vi "XYZ_XYStage.vi"(0 "command":string, 5 "XY details":string, 7 "VISA Write_Read":T1={"VISA resource name"="", "instrument model"="XY-STAGE:MODEL", "command array"=[], "command terminator"="\r", "expected reply"="\r", "reply terminator"="\r", "numeric array out"=[], "string array out"=[]}, 11 "Error in (no error)":errorcluster) -> (4 "x":dbl, 6 "y":dbl, 8 "Success":bool, 10 "VISA Write_Read out":T1={"VISA resource name"="", "instrument model"="XY-STAGE:MODEL", "command array"=[], "command terminator"="\r", "expected reply"="\r", "reply terminator"="\r", "numeric array out"=[], "string array out"=[]}, 15 "Error out":errorcluster)   [LabVIEW 2013]
uses:
  TypeDef VISA Write_Read.ctl
  <vilib>/Instr/_visa.llb/VISA Flush IO Buffer Mask.ctl
  Global.vi
  <vilib>/Instr/_visa.llb/VISA Configure Serial Port (Instr).vi
panel:
  in  "VISA Connection":T3={"enable termination char"=TRUE, "termination char"=10, "timeout"=10000, "VISA resource name"="", "baud rate"=9600, "data bits"=8, "parity"=enum."None", "stop bits"=10, "flow control"=0, "mask array"=[]} {"mask array" items=["Flush Receive Buffer"=16, "Write Transmit Buffer to Device"=32, "Flush Receive Buffer (No I/O)"=64, "Flush Transmit Buffer"=128]; "flow control" items=["None", "XON/XOFF", "RTS/CTS", "XON/XOFF & RTS/CTS", "DTR/DSR", "XON/XOFF & DTR/DSR"]; "stop bits" items=["1.0"=10, "1.5"=15, "2.0"=20]; "data bits" min=5 max=8 step=1; "termination char" format="%.0x"}
  in  "delay":u32=200
  in  "timeout":i32=10000
  out "Sbytes out":i32
  out "Sreply":string
  out "Dbytes out":u32
  out "Dreply":string
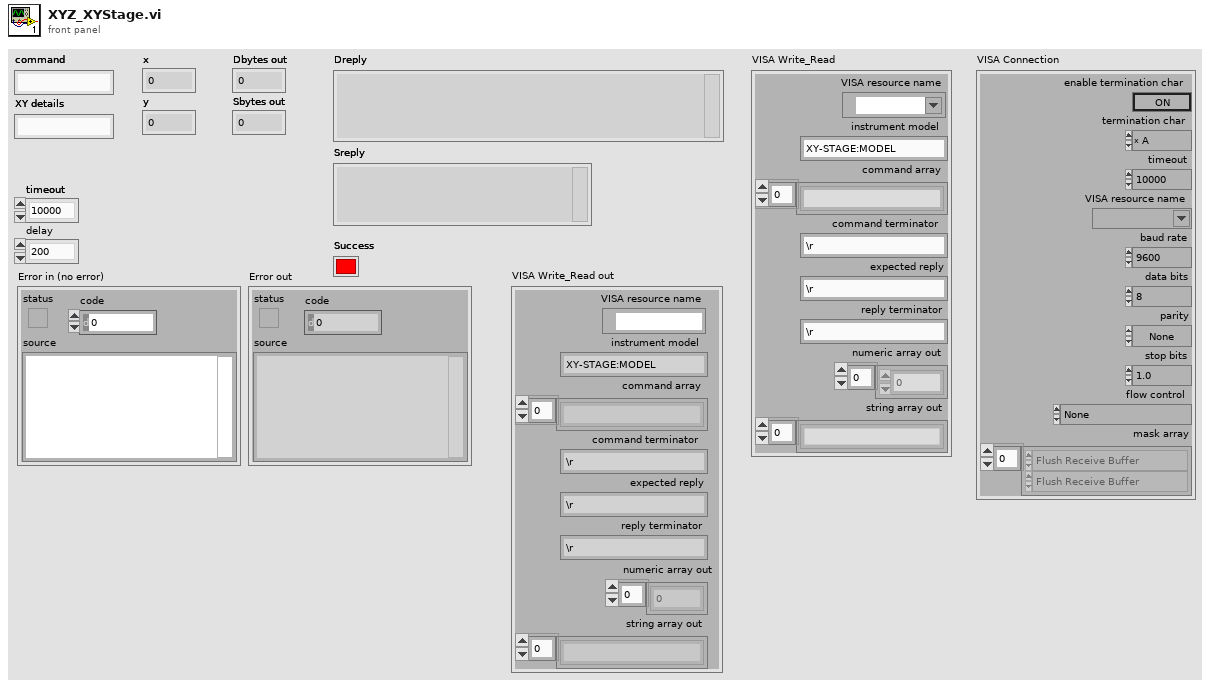
[diagram p1: front panel]
types:
  T1 = typedef "TypeDef VISA Write_Read.ctl" = cluster{"VISA resource name":refnum<visa-resource-name>, "instrument model":string, "command array":string[], "command terminator":string, "expected reply":string, "reply terminator":string, "numeric array out":dbl[], "string array out":string[]}
  T2 = typedef "VISA Flush IO Buffer Mask.ctl" = u16
  T3 = cluster{"enable termination char":bool, "termination char":u8, "timeout":u32, "VISA resource name":refnum<visa-resource-name>, "baud rate":u32, "data bits":u16, "parity":enum16{"None", "Odd", "Even", "Mark", "Space"}, "stop bits":u16, "flow control":u16, "mask array":T2[]}
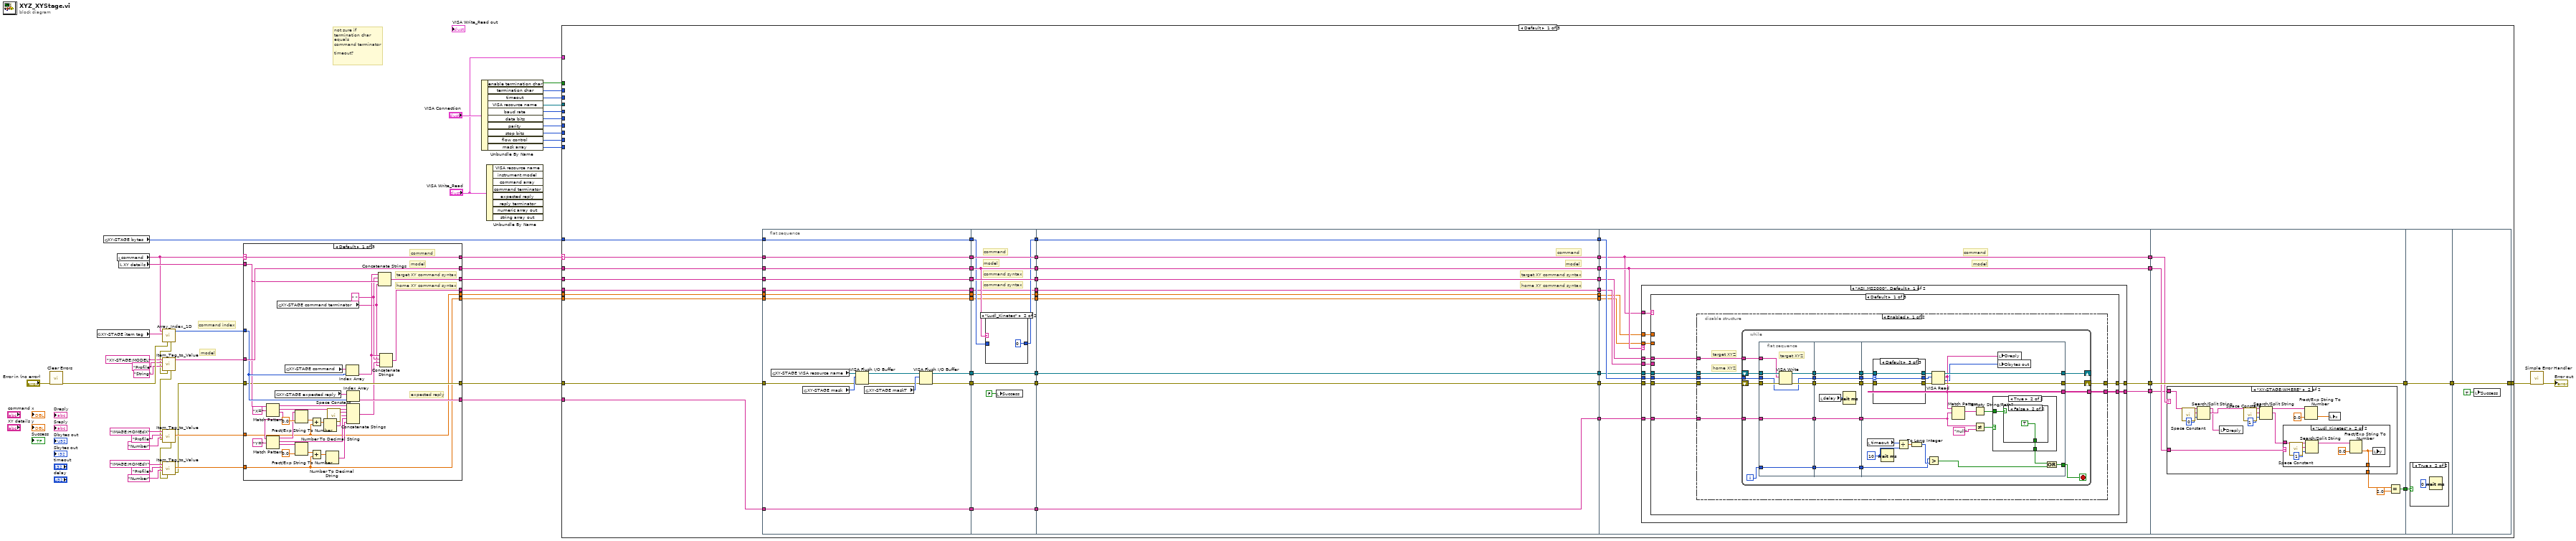
[diagram p0: block diagram]
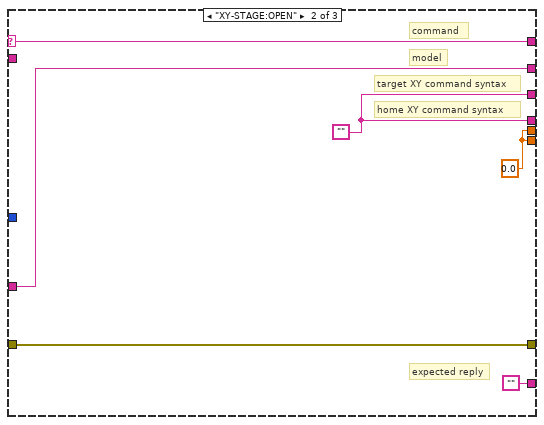
[diagram p2: hidden frame]
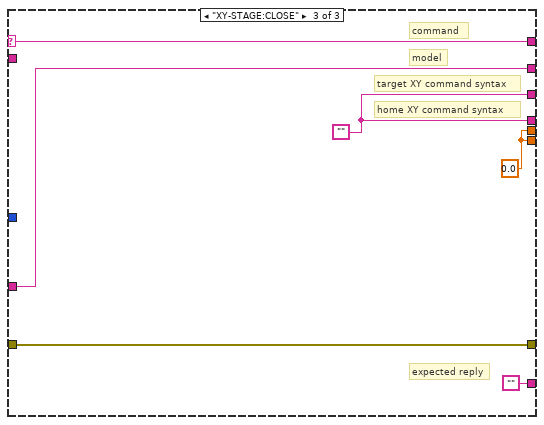
[diagram p3: hidden frame]
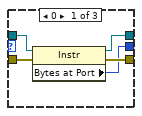
[diagram p5: hidden frame]
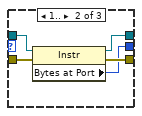
[diagram p6: hidden frame]
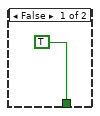
[diagram p7: hidden frame]
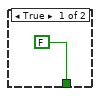
[diagram p8: hidden frame]
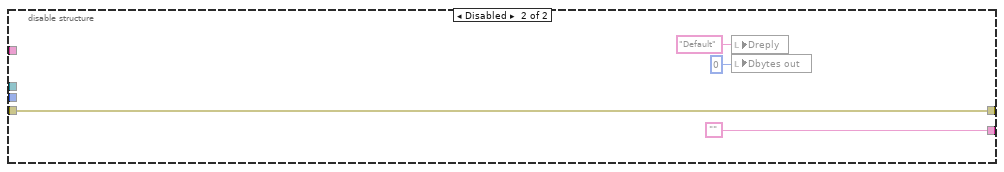
[diagram p9: hidden frame]
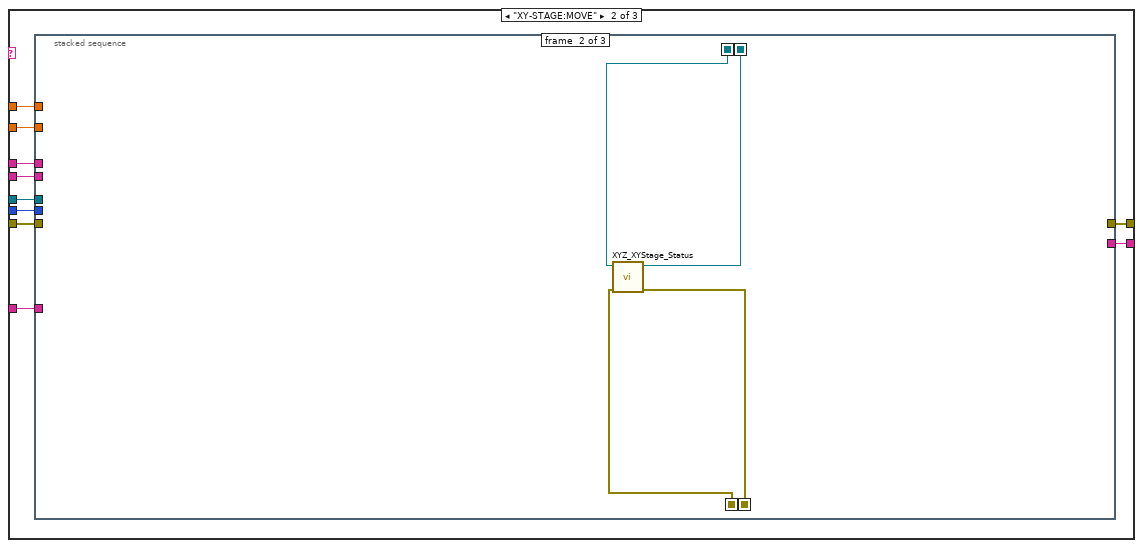
[diagram p10: hidden frame]
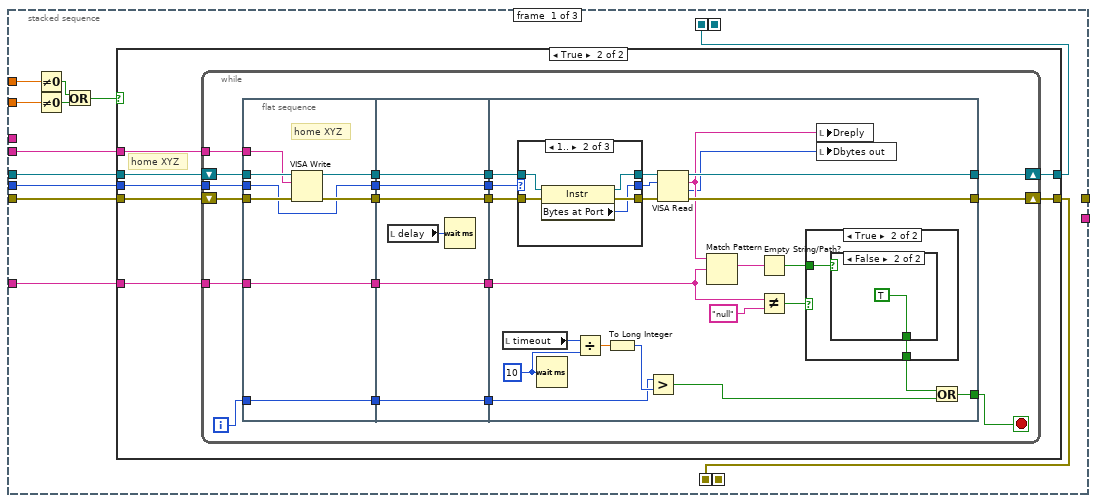
[diagram p11: hidden frame]
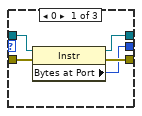
[diagram p13: hidden frame]
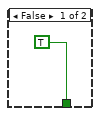
[diagram p15: hidden frame]
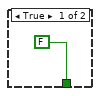
[diagram p16: hidden frame]
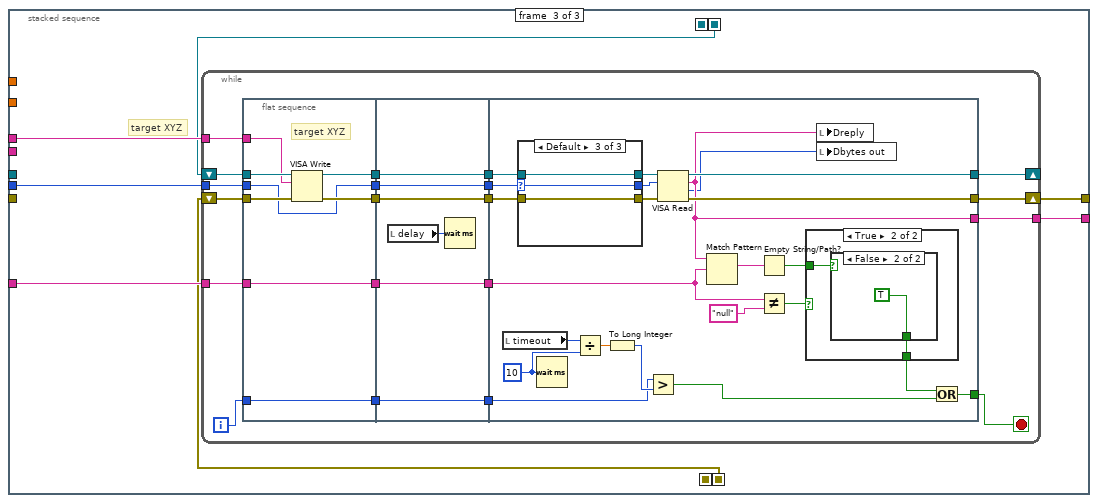
[diagram p17: hidden frame]
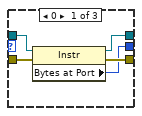
[diagram p18: hidden frame]
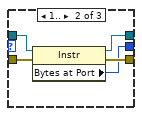
[diagram p19: hidden frame]
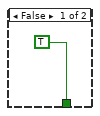
[diagram p20: hidden frame]
diagram:
  # "not sure if \ntermination char\nequals\ncommand terminator\n\ntimeout?"
  # "model"
  # "command index"
  n1 = call <vilib>:"Clear Errors.vi"("error in (no error)"="Error in (no error)") -> ("error out"=w43:errorcluster)  [unwired: 6 in]
  n2 = global read "Global.vi" "XY-STAGE item tag"() -> (w31:string[])
  n3 = global read "Global.vi" "XY-STAGE bytes"() -> (w27:u32)
  n4 = local read "command"() -> (w30:string)
  n5 = local read "XY details"() -> (w40:string)
  n6 = call "Array_Index_1D.vi"("Error in (no error)"=w43, "Array"=w31, "Element string"=w30) -> ("Array row"=w29:i32, "Error out"=w28:errorcluster)  [unwired: 7 in]
  n7 = call "Item_Tag_to_Value.vi"("Error in (no error)"=w28, "Value Mode"="String", "Value Source"="Profile", "Item Tag"="XY-STAGE:MODEL" ("regular expression")) -> ("Output String"=w33:string, "Error out"=w17:errorcluster)  [unwired: 3 in, 3 out]
  n8 = call "Item_Tag_to_Value.vi"("Error in (no error)"=w17, "Value Mode"="Number", "Value Source"="Profile", "Item Tag"="IMAGE:HOMEdX" ("regular expression")) -> ("Output Number"=w19:dbl, "Error out"=w18:errorcluster)  [unwired: 3 in, 3 out]
  n9 = call "Item_Tag_to_Value.vi"("Error in (no error)"=w18, "Value Mode"="Number", "Value Source"="Profile", "Item Tag"="IMAGE:HOMEdY" ("regular expression")) -> ("Output Number"=w20:dbl, "Error out"=w16:errorcluster)  [unwired: 3 in, 3 out]
  n10 = case shown="Default" w30 {
    selector: w30 -> [w76 w84 w90]
    tunnel: [w76 w84 w90] -> w41
    tunnel: w40 -> [w63 _ _]
    tunnel: [w75 w80 w86] -> w38
    tunnel: [w53 "" ("String") "" ("String")] -> w39
    tunnel: [w74 w83 w89] -> w37
    tunnel: w33 -> [w74 w83 w89]
    tunnel: w16 -> [w54 w82 w88]
    tunnel: [w54 w82 w88] -> w32
    tunnel: w29 -> [w73 _ _]
    tunnel: w20 -> [w46 _ _]
    tunnel: w19 -> [w47 _ _]
    tunnel: [w48 w80 w86] -> w15
    tunnel: [w47 w79 w85] -> w14
    tunnel: [w46 w79 w85] -> w13
    frame Default {
      w51 = " " ("string")
      # "home XY command syntax"
      # "target XY command syntax"
      # "command"
      # "model"
      # "expected reply"
      n11 = Match Pattern(string=w63, regular expression="X=") -> (before substring=w60:string, match substring=w59:string, after substring=w61:string)  [unwired: 1 in, 1 out]
      n12 = Match Pattern(string=w61, regular expression="Y=") -> (before substring=w62:string, match substring=w56:string, after substring=w67:string)  [unwired: 1 in, 1 out]
      n13 = global read "Global.vi" "XY-STAGE expected reply"() -> (w77:string[])
      n14 = global read "Global.vi" "XY-STAGE command terminator"() -> (w49:string)
      n15 = global read "Global.vi" "XY-STAGE command"() -> (w78:string[])
      n16 = Fract/Exp String To Number(string=w62, default (0 dbl)=0.0 ("default (0 DBL)")) -> (number=w70:dbl)  [unwired: 2 in, 1 out]
      n17 = Fract/Exp String To Number(string=w67, default (0 dbl)=0.0 ("default (0 DBL)")) -> (number=w65:dbl)  [unwired: 2 in, 1 out]
      n18 = Add(x=w70, y=w47) -> (x+y=w69:dbl)
      n19 = Add(x=w65, y=w46) -> (x+y=w64:dbl)
      n20 = Number To Decimal String(number=w69) -> (decimal integer string=w58:string)  [unwired: 1 in]
      n21 = Number To Decimal String(number=w64) -> (decimal integer string=w55:string)  [unwired: 1 in]
      n22 = call <vilib>:"Space Constant.vi"() -> ("String"=w57:string)
      n23 = Index Array(array=w78, index=w73) -> (element=w52:string)
      n24 = Index Array(array=w77, index=w73) -> (element=w53:string)
      n25 = Concatenate Strings(w60, w59, w58, w57, w56, w55) -> (w50:string)
      n26 = Concatenate Strings(w52, w51, w63, w49) -> (w75:string)
      n27 = Concatenate Strings(w52, w51, w50, w49) -> (w48:string)
    }
    frame "XY-STAGE:OPEN" {
      w79 = 0.0 ("Output Number")
      w80 = ""
      # "home XY command syntax"
      # "target XY command syntax"
      # "command"
      # "model"
      # "expected reply"
    }
    frame "XY-STAGE:CLOSE" {
      w85 = 0.0 ("Output Number")
      w86 = ""
      # "home XY command syntax"
      # "target XY command syntax"
      # "command"
      # "model"
      # "expected reply"
    }
  }
  n28 = Unbundle By Name("VISA Connection") -> ("enable termination char"=w12:bool, "termination char"=w11:u8, "timeout"=w10:u32, "VISA resource name"=w9:refnum<visa-resource-name>, "baud rate"=w8:u32, "data bits"=w7:u16, "parity"=w6:enum16{"None", "Odd", "Even", "Mark", "Space"}, "stop bits"=w5:u16, "flow control"=w4:u16, "mask array"=w3:T2[])
  n29 = Unbundle By Name("VISA Write_Read") -> ()  [unwired: 8 out]
  n30 = case shown="Default" w41 {
    selector: w41 -> [w135 _ _]
    tunnel: w39 -> [w137 _ _]
    tunnel: w38 -> [w117 _ _]
    tunnel: w37 -> [w136 w983 w1026]
    tunnel: w32 -> [w109 w985 w1028]
    tunnel: [w133 w984 w1027] -> w45
    tunnel: w27 -> [w107 _ _]
    tunnel: w15 -> [w103 _ _]
    tunnel: w14 -> [w100 _ _]
    tunnel: w13 -> [w99 _ _]
    tunnel: w12 -> [_ _ w1021]
    tunnel: w11 -> [_ _ w1019]
    tunnel: w10 -> [_ _ w1017]
    tunnel: w9 -> [_ _ w1015]
    tunnel: w8 -> [_ _ w1013]
    tunnel: w7 -> [_ _ w1011]
    tunnel: w6 -> [_ _ w1009]
    tunnel: w5 -> [_ _ w1007]
    tunnel: w4 -> [_ _ w1005]
    tunnel: w3 -> [_ _ w1003]
    tunnel: "VISA Write_Read" -> [_ _ _]
    frame Default {
      n31 = flat-sequence {
        tunnel: w117 -> [w150]
        tunnel: w135 -> [w151]
        tunnel: w137 -> [w152]
        tunnel: w136 -> [w153]
        tunnel: w109 -> [w144]
        tunnel: [w143] -> w114
        tunnel: [w153] -> w113
        tunnel: [w152] -> w112
        tunnel: [w151] -> w111
        tunnel: [w150] -> w110
        tunnel: [w142] -> w108
        tunnel: w107 -> [w141]
        tunnel: [w141] -> w105
        tunnel: w103 -> [w140]
        tunnel: [w140] -> w101
        tunnel: w100 -> [w139]
        tunnel: w99 -> [w138]
        tunnel: [w139] -> w97
        tunnel: [w138] -> w95
        tunnel: [w165] -> w127
        tunnel: [w159] -> w125
        tunnel: [w164] -> w123
        tunnel: [w162] -> w121
        tunnel: [w161] -> w119
        tunnel: [w160] -> w116
        tunnel: w114 -> [w161]
        tunnel: w113 -> [w159]
        tunnel: w112 -> [w165]
        tunnel: w111 -> [w164]
        tunnel: w110 -> [w160]
        tunnel: w108 -> [w162]
        tunnel: [w157] -> w106
        tunnel: w105 -> [w158]
        tunnel: [w156] -> w102
        tunnel: w101 -> [w156]
        tunnel: [w155] -> w98
        tunnel: w97 -> [w155]
        tunnel: [w154] -> w96
        tunnel: w95 -> [w154]
        tunnel: w127 -> [w177]
        tunnel: [w177] -> w126
        tunnel: w125 -> [w174]
        tunnel: [w174] -> w124
        tunnel: w123 -> [w176]
        tunnel: [w176] -> w122
        tunnel: w121 -> [w172]
        tunnel: [w172] -> w120
        tunnel: w119 -> [w171]
        tunnel: [w171] -> w118
        tunnel: w116 -> [w175]
        tunnel: [w175] -> w115
        tunnel: w106 -> [w173]
        tunnel: [w173] -> w104
        tunnel: w102 -> [w170]
        tunnel: w98 -> [w169]
        tunnel: w96 -> [w168]
        tunnel: [w170] -> w94
        tunnel: [w169] -> w93
        tunnel: [w168] -> w92
        tunnel: w126 -> [w188]
        tunnel: w124 -> [w187]
        tunnel: [w189] -> w132
        tunnel: [w187] -> w131
        tunnel: [w184] -> w130
        tunnel: w122 -> [w184]
        tunnel: w120 -> [w178]
        tunnel: w118 -> [w179]
        tunnel: [w186] -> w129
        tunnel: w115 -> [w182]
        tunnel: w104 -> [w185]
        tunnel: w94 -> [w183]
        tunnel: w93 -> [w181]
        tunnel: w92 -> [w180]
        tunnel: [w950] -> w134
        tunnel: w129 -> [w947]
        tunnel: w130 -> [w948]
        tunnel: w131 -> [w949]
        tunnel: w132 -> [w950]
        tunnel: [w944] -> w91
        tunnel: w134 -> [w976]
        tunnel: [w976] -> w128
        tunnel: w91 -> [w975]
        tunnel: [w979] -> w133
        tunnel: w128 -> [w979]
        frame #0 {
          n32 = global read "Global.vi" "XY-STAGE VISA resource name"() -> (w145:refnum<visa-resource-name>)
          n33 = global read "Global.vi" "XY-STAGE mask"() -> (w146:u16)
          n34 = VISA Flush I/O Buffer(VISA resource name=w145, mask (16)=w146, error in (no error)=w144) -> (VISA resource name out=w148:refnum<visa-resource-name>, error out=w147:errorcluster)
          n35 = global read "Global.vi" "XY-STAGE maskT"() -> (w149:u16)
          n36 = VISA Flush I/O Buffer(VISA resource name=w148, mask (16)=w149, error in (no error)=w147) -> (VISA resource name out=w142:refnum<visa-resource-name>, error out=w143:errorcluster)
        }
        frame #1 {
          # "command syntax"
          # "command syntax"
          # "model"
          # "command"
          n37 = case shown="\"Ludl_Kinetec\"" w159 {
            tunnel: w158 -> [w166 _]
            tunnel: [w166 u32 0 ("XY-STAGE bytes")] -> w157
            frame "ASI_MS2000", Default {
            }
            frame "Ludl_Kinetec" {
            }
          }
          n38 = local write "Success"(FALSE ("Success")) -> ()
        }
        frame #2 {
          # "home XY command syntax"
          # "target XY command syntax"
          # "command"
          # "model"
        }
        frame #3 {
          # "command"
          # "model"
          n39 = case shown="\"ASI_MS2000\", Default" w187 {
            tunnel: [w200 w577] -> w189
            tunnel: w188 -> [w199 w576]
            tunnel: w178 -> [w198 w575]
            tunnel: w179 -> [w197 w574]
            tunnel: [w196 w573] -> w186
            tunnel: w185 -> [w195 w572]
            tunnel: w184 -> [w194 w571]
            tunnel: w183 -> [w193 w570]
            tunnel: w182 -> [w192 w569]
            tunnel: w181 -> [w191 w568]
            tunnel: w180 -> [w190 w567]
            frame "ASI_MS2000", Default {
              n40 = case shown="Default" w194 {
                tunnel: [w202 w298 w486] -> w200
                tunnel: w199 -> [w203 w299 w487]
                tunnel: w198 -> [w206 w302 w490]
                tunnel: w197 -> [w204 w300 w488]
                tunnel: [w201 w297 w485] -> w196
                tunnel: w195 -> [w205 w301 w489]
                tunnel: w193 -> [_ w294 _]
                tunnel: w192 -> [w207 w303 w491]
                tunnel: w191 -> [_ w296 _]
                tunnel: w190 -> [_ w295 _]
                frame Default {
                  n41 = disable-structure shown="Enabled" {
                    disable-tunnel: w207 -> [w214 _]
                    disable-tunnel: w206 -> [w213 _]
                    disable-tunnel: w205 -> [w212 _]
                    disable-tunnel: w204 -> [w211 w293]
                    disable-tunnel: w203 -> [w210 _]
                    disable-tunnel: [w209 w293] -> w202
                    disable-tunnel: [w208 "" ("read buffer")] -> w201
                    frame Enabled {
                      # "home XYZ"
                      # "target XYZ"
                      n42 = while {
                        shift-right: [w223] -> _
                        shift-left: w213 -> [w221]
                        shift-right: [w224] -> w209
                        shift-left: w211 -> [w219]
                        tunnel: w210 -> [w218]
                        tunnel: [w225] -> w208
                        tunnel: w214 -> [w222]
                        tunnel: w212 -> [w220]
                        i -> [w217]
                        stop <- w226 stop-if-true
                        n43 = flat-sequence {
                          tunnel: w221 -> [w239]
                          tunnel: w219 -> [w240]
                          tunnel: w218 -> [w242]
                          tunnel: [w242] -> w234
                          tunnel: [w236] -> w233
                          tunnel: [w237] -> w232
                          tunnel: [w241] -> w231
                          tunnel: w222 -> [w238]
                          tunnel: w220 -> [w237]
                          tunnel: w217 -> [w235]
                          tunnel: [w235] -> w215
                          tunnel: [w248] -> w230
                          tunnel: [w247] -> w229
                          tunnel: [w246] -> w228
                          tunnel: [w245] -> w227
                          tunnel: w234 -> [w248]
                          tunnel: w233 -> [w246]
                          tunnel: w232 -> [w245]
                          tunnel: w231 -> [w247]
                          tunnel: [w243] -> w216
                          tunnel: w215 -> [w243]
                          tunnel: [w269] -> w223
                          tunnel: [w268] -> w224
                          tunnel: [w250] -> w225
                          tunnel: w230 -> [w252]
                          tunnel: w229 -> [w261]
                          tunnel: w228 -> [w260]
                          tunnel: w227 -> [w256]
                          tunnel: [w255] -> w226
                          tunnel: w216 -> [w254]
                          frame #0 {
                            # "target XYZ"
                            n44 = VISA Write(VISA resource name=w239, write buffer=w238, error in (no error)=w240) -> (VISA resource name out=w236:refnum<visa-resource-name>, error out=w241:errorcluster)  [unwired: 1 out]
                          }
                          frame #1 {
                            n45 = local read "delay"() -> (w244:u32)
                            n46 = Wait (ms)(milliseconds to wait=w244) -> ()  [unwired: 1 out]
                          }
                          frame #2 {
                            w267 = u32 10 ("milliseconds to wait")
                            n47 = local read "timeout"() -> (w262:i32)
                            n48 = case shown="Default" w256 {
                              selector: w256 -> [_ _ w284]
                              tunnel: [w276 w281 w282] -> w257
                              tunnel: [w275 w280 w283] -> w259
                              tunnel: [w274 w279 w284] -> w258
                              tunnel: w260 -> [w273 w278 w283]
                              tunnel: w261 -> [w272 w277 w282]
                              frame 0 {
                                n49 = property class="Instr"(reference=w273, error in=w272) -> (reference out=w275:refnum<visa-resource-name>, error out=w276:errorcluster, "Bytes at Port"=w274:u32)
                              }
                              frame 1.. {
                                n50 = property class="Instr"(reference=w278, error in=w277) -> (reference out=w280:refnum<visa-resource-name>, error out=w281:errorcluster, "Bytes at Port"=w279:u32)
                              }
                              frame Default {
                              }
                            }
                            n51 = Wait (ms)(milliseconds to wait=w267) -> ()  [unwired: 1 out]
                            n52 = Divide(x=w262, y=w267) -> (x/y=w266:dbl)
                            n53 = To Long Integer(number=w266) -> (32bit integer=w265:i32)
                            n54 = Greater?(x=w254, y=w265) -> (0:w264:bool)
                            n55 = VISA Read(VISA resource name=w259, byte count=w258, error in (no error)=w257) -> (VISA resource name out=w269:refnum<visa-resource-name>, read buffer=w250:string, return count=w249:u32, error out=w268:errorcluster)
                            n56 = Match Pattern(string=w250, regular expression=w252) -> (match substring=w251:string)  [unwired: 1 in, 3 out]
                            n57 = Empty String/Path?(string/path=w251) -> (empty?=w253:bool)
                            n58 = Not Equal?(x=w252, y="null") -> (x != y?=w270:bool)
                            n59 = case shown="True" w270 {
                              tunnel: [TRUE w286] -> w263
                              tunnel: w253 -> [_ w287]
                              frame False {
                              }
                              frame True {
                                n60 = case shown="False" w287 {
                                tunnel: [FALSE TRUE] -> w286
                                frame True {
                                }
                                frame False {
                                }
                                }
                              }
                            }
                            n61 = local write "Dreply"(w250) -> ()
                            n62 = local write "Dbytes out"(w249) -> ()
                            n63 = Or(x=w263, y=w264) -> (x .or. y?=w255:bool)
                          }
                        }
                      }
                    }
                    frame Disabled {
                      n64 = local write "Dreply"("Default" ("Dreply")) -> ()
                      n65 = local write "Dbytes out"(u32 0 ("Dbytes out")) -> ()
                    }
                  }
                }
                frame "XY-STAGE:MOVE" {
                  n66 = stacked-sequence {
                    seq-local: [w304 _ _] -> [_ w402 _]
                    seq-local: [_ w401 _] -> [_ _ w405]
                    seq-local: [w305 _ _] -> [_ w400 _]
                    seq-local: [_ w399 _] -> [_ _ w403]
                    tunnel: w303 -> [_ _ w409]
                    tunnel: w302 -> [w315 _ _]
                    tunnel: w301 -> [w314 _ w408]
                    tunnel: w300 -> [w313 _ _]
                    tunnel: w299 -> [w312 _ w407]
                    tunnel: [_ _ w404] -> w298
                    tunnel: [_ _ w406] -> w297
                    tunnel: w296 -> [w309 _ _]
                    tunnel: w295 -> [w308 _ _]
                    tunnel: w294 -> [w306 _ _]
                    frame #0 {
                      n67 = Not Equal To 0?(x=w309) -> (x != 0?=w311:bool)
                      n68 = Not Equal To 0?(x=w308) -> (x != 0?=w310:bool)
                      n69 = Or(x=w311, y=w310) -> (x .or. y?=w307:bool)
                      n70 = case shown="True" w307 {
                        tunnel: w315 -> [w317 w324]
                        tunnel: w314 -> [_ w323]
                        tunnel: w313 -> [w316 w322]
                        tunnel: w312 -> [_ w321]
                        tunnel: [w316 w320] -> w305
                        tunnel: w306 -> [_ w319]
                        tunnel: [w317 w318] -> w304
                        frame False {
                        }
                        frame True {
                          # "home XYZ"
                          n71 = while {
                            shift-right: [w333] -> w318
                            shift-left: w324 -> [w332]
                            shift-right: [w334] -> w320
                            shift-left: w322 -> [w330]
                            tunnel: w321 -> [w329]
                            tunnel: w323 -> [w331]
                            tunnel: w319 -> [w325]
                            i -> [w328]
                            stop <- w335 stop-if-true
                            n72 = flat-sequence {
                              tunnel: w332 -> [w348]
                              tunnel: w330 -> [w349]
                              tunnel: w329 -> [w351]
                              tunnel: [w351] -> w343
                              tunnel: [w346] -> w342
                              tunnel: [w347] -> w341
                              tunnel: [w350] -> w340
                              tunnel: w331 -> [w347]
                              tunnel: w328 -> [w345]
                              tunnel: [w345] -> w326
                              tunnel: w325 -> [w344]
                              tunnel: [w357] -> w339
                              tunnel: [w356] -> w338
                              tunnel: [w355] -> w337
                              tunnel: [w354] -> w336
                              tunnel: w343 -> [w357]
                              tunnel: w342 -> [w355]
                              tunnel: w341 -> [w354]
                              tunnel: w340 -> [w356]
                              tunnel: [w352] -> w327
                              tunnel: w326 -> [w352]
                              tunnel: [w378] -> w333
                              tunnel: [w377] -> w334
                              tunnel: w339 -> [w361]
                              tunnel: w338 -> [w370]
                              tunnel: w337 -> [w369]
                              tunnel: w336 -> [w365]
                              tunnel: [w364] -> w335
                              tunnel: w327 -> [w363]
                              frame #0 {
                                # "home XYZ"
                                n73 = VISA Write(VISA resource name=w348, write buffer=w344, error in (no error)=w349) -> (VISA resource name out=w346:refnum<visa-resource-name>, error out=w350:errorcluster)  [unwired: 1 out]
                              }
                              frame #1 {
                                n74 = local read "delay"() -> (w353:u32)
                                n75 = Wait (ms)(milliseconds to wait=w353) -> ()  [unwired: 1 out]
                              }
                              frame #2 {
                                w376 = u32 10 ("milliseconds to wait")
                                n76 = local read "timeout"() -> (w371:i32)
                                n77 = case shown="1.." w365 {
                                selector: w365 -> [_ _ w393]
                                tunnel: [w385 w390 w391] -> w366
                                tunnel: [w384 w389 w392] -> w368
                                tunnel: [w383 w388 w393] -> w367
                                tunnel: w369 -> [w382 w387 w392]
                                tunnel: w370 -> [w381 w386 w391]
                                frame 0 {
                                n78 = property class="Instr"(reference=w382, error in=w381) -> (reference out=w384:refnum<visa-resource-name>, error out=w385:errorcluster, "Bytes at Port"=w383:u32)
                                }
                                frame 1.. {
                                n79 = property class="Instr"(reference=w387, error in=w386) -> (reference out=w389:refnum<visa-resource-name>, error out=w390:errorcluster, "Bytes at Port"=w388:u32)
                                }
                                frame Default {
                                }
                                }
                                n80 = Wait (ms)(milliseconds to wait=w376) -> ()  [unwired: 1 out]
                                n81 = Divide(x=w371, y=w376) -> (x/y=w375:dbl)
                                n82 = To Long Integer(number=w375) -> (32bit integer=w374:i32)
                                n83 = Greater?(x=w363, y=w374) -> (0:w373:bool)
                                n84 = VISA Read(VISA resource name=w368, byte count=w367, error in (no error)=w366) -> (VISA resource name out=w378:refnum<visa-resource-name>, read buffer=w359:string, return count=w358:u32, error out=w377:errorcluster)
                                n85 = Match Pattern(string=w359, regular expression=w361) -> (match substring=w360:string)  [unwired: 1 in, 3 out]
                                n86 = Empty String/Path?(string/path=w360) -> (empty?=w362:bool)
                                n87 = Not Equal?(x=w361, y="null") -> (x != y?=w379:bool)
                                n88 = case shown="True" w379 {
                                tunnel: [TRUE w395] -> w372
                                tunnel: w362 -> [_ w396]
                                frame False {
                                }
                                frame True {
                                n89 = case shown="False" w396 {
                                tunnel: [FALSE TRUE] -> w395
                                frame True {
                                }
                                frame False {
                                }
                                }
                                }
                                }
                                n90 = local write "Dreply"(w359) -> ()
                                n91 = local write "Dbytes out"(w358) -> ()
                                n92 = Or(x=w372, y=w373) -> (x .or. y?=w364:bool)
                              }
                            }
                          }
                        }
                      }
                    }
                    frame #1 {
                      n93 = call "XYZ_XYStage_Status.vi"("error in (no error)"=w400, "VISA resource name"=w402) -> ("error out"=w399:errorcluster, "VISA resource name out"=w401:refnum<visa-resource-name>)  [unwired: 4 in, 1 out]
                    }
                    frame #2 {
                      # "target XYZ"
                      n94 = while {
                        shift-right: [w418] -> _
                        shift-left: w405 -> [w416]
                        shift-right: [w419] -> w404
                        shift-left: w403 -> [w414]
                        tunnel: w407 -> [w413]
                        tunnel: [w420] -> w406
                        tunnel: w409 -> [w417]
                        tunnel: w408 -> [w415]
                        i -> [w412]
                        stop <- w421 stop-if-true
                        n95 = flat-sequence {
                          tunnel: w416 -> [w434]
                          tunnel: w414 -> [w435]
                          tunnel: w413 -> [w437]
                          tunnel: [w437] -> w429
                          tunnel: [w432] -> w428
                          tunnel: [w433] -> w427
                          tunnel: [w436] -> w426
                          tunnel: w417 -> [w430]
                          tunnel: w415 -> [w433]
                          tunnel: w412 -> [w431]
                          tunnel: [w431] -> w410
                          tunnel: [w443] -> w425
                          tunnel: [w442] -> w424
                          tunnel: [w441] -> w423
                          tunnel: [w440] -> w422
                          tunnel: w429 -> [w443]
                          tunnel: w428 -> [w441]
                          tunnel: w427 -> [w440]
                          tunnel: w426 -> [w442]
                          tunnel: [w438] -> w411
                          tunnel: w410 -> [w438]
                          tunnel: [w464] -> w418
                          tunnel: [w463] -> w419
                          tunnel: [w445] -> w420
                          tunnel: w425 -> [w447]
                          tunnel: w424 -> [w456]
                          tunnel: w423 -> [w455]
                          tunnel: w422 -> [w451]
                          tunnel: [w450] -> w421
                          tunnel: w411 -> [w449]
                          frame #0 {
                            # "target XYZ"
                            n96 = VISA Write(VISA resource name=w434, write buffer=w430, error in (no error)=w435) -> (VISA resource name out=w432:refnum<visa-resource-name>, error out=w436:errorcluster)  [unwired: 1 out]
                          }
                          frame #1 {
                            n97 = local read "delay"() -> (w439:u32)
                            n98 = Wait (ms)(milliseconds to wait=w439) -> ()  [unwired: 1 out]
                          }
                          frame #2 {
                            w462 = u32 10 ("milliseconds to wait")
                            n99 = local read "timeout"() -> (w457:i32)
                            n100 = case shown="Default" w451 {
                              selector: w451 -> [_ _ w479]
                              tunnel: [w471 w476 w477] -> w452
                              tunnel: [w470 w475 w478] -> w454
                              tunnel: [w469 w474 w479] -> w453
                              tunnel: w455 -> [w468 w473 w478]
                              tunnel: w456 -> [w467 w472 w477]
                              frame 0 {
                                n101 = property class="Instr"(reference=w468, error in=w467) -> (reference out=w470:refnum<visa-resource-name>, error out=w471:errorcluster, "Bytes at Port"=w469:u32)
                              }
                              frame 1.. {
                                n102 = property class="Instr"(reference=w473, error in=w472) -> (reference out=w475:refnum<visa-resource-name>, error out=w476:errorcluster, "Bytes at Port"=w474:u32)
                              }
                              frame Default {
                              }
                            }
                            n103 = Wait (ms)(milliseconds to wait=w462) -> ()  [unwired: 1 out]
                            n104 = Divide(x=w457, y=w462) -> (x/y=w461:dbl)
                            n105 = To Long Integer(number=w461) -> (32bit integer=w460:i32)
                            n106 = Greater?(x=w449, y=w460) -> (0:w459:bool)
                            n107 = VISA Read(VISA resource name=w454, byte count=w453, error in (no error)=w452) -> (VISA resource name out=w464:refnum<visa-resource-name>, read buffer=w445:string, return count=w444:u32, error out=w463:errorcluster)
                            n108 = Match Pattern(string=w445, regular expression=w447) -> (match substring=w446:string)  [unwired: 1 in, 3 out]
                            n109 = Empty String/Path?(string/path=w446) -> (empty?=w448:bool)
                            n110 = Not Equal?(x=w447, y="null") -> (x != y?=w465:bool)
                            n111 = case shown="True" w465 {
                              tunnel: [TRUE w481] -> w458
                              tunnel: w448 -> [_ w482]
                              frame False {
                              }
                              frame True {
                                n112 = case shown="False" w482 {
                                tunnel: [FALSE TRUE] -> w481
                                frame True {
                                }
                                frame False {
                                }
                                }
                              }
                            }
                            n113 = local write "Dreply"(w445) -> ()
                            n114 = local write "Dbytes out"(w444) -> ()
                            n115 = Or(x=w458, y=w459) -> (x .or. y?=w450:bool)
                          }
                        }
                      }
                    }
                  }
                }
                frame "XY-STAGE:STATUS" {
                  # "home XYZ"
                  # "target XYZ"
                  n116 = while {
                    shift-right: [w500] -> _
                    shift-left: w490 -> [w498]
                    shift-right: [w501] -> w486
                    shift-left: w488 -> [w496]
                    tunnel: w487 -> [w495]
                    tunnel: [w502] -> w485
                    tunnel: w491 -> [w499]
                    tunnel: w489 -> [w497]
                    i -> [w494]
                    stop <- w503 stop-if-true
                    n117 = flat-sequence {
                      tunnel: w498 -> [w516]
                      tunnel: w496 -> [w517]
                      tunnel: w495 -> [w519]
                      tunnel: [w519] -> w511
                      tunnel: [w513] -> w510
                      tunnel: [w514] -> w509
                      tunnel: [w518] -> w508
                      tunnel: w499 -> [w515]
                      tunnel: w497 -> [w514]
                      tunnel: w494 -> [w512]
                      tunnel: [w512] -> w492
                      tunnel: [w525] -> w507
                      tunnel: [w524] -> w506
                      tunnel: [w523] -> w505
                      tunnel: [w522] -> w504
                      tunnel: w511 -> [w525]
                      tunnel: w510 -> [w523]
                      tunnel: w509 -> [w522]
                      tunnel: w508 -> [w524]
                      tunnel: [w520] -> w493
                      tunnel: w492 -> [w520]
                      tunnel: [w546] -> w500
                      tunnel: [w545] -> w501
                      tunnel: [w527] -> w502
                      tunnel: w507 -> [w529]
                      tunnel: w506 -> [w538]
                      tunnel: w505 -> [w537]
                      tunnel: w504 -> [w533]
                      tunnel: [w532] -> w503
                      tunnel: w493 -> [w531]
                      frame #0 {
                        # "target XYZ"
                        n118 = VISA Write(VISA resource name=w516, write buffer=w515, error in (no error)=w517) -> (VISA resource name out=w513:refnum<visa-resource-name>, error out=w518:errorcluster)  [unwired: 1 out]
                      }
                      frame #1 {
                        n119 = local read "delay"() -> (w521:u32)
                        n120 = Wait (ms)(milliseconds to wait=w521) -> ()  [unwired: 1 out]
                      }
                      frame #2 {
                        w544 = u32 10 ("milliseconds to wait")
                        n121 = local read "timeout"() -> (w539:i32)
                        n122 = case shown="Default" w533 {
                          selector: w533 -> [_ _ w561]
                          tunnel: [w553 w558 w559] -> w534
                          tunnel: [w552 w557 w560] -> w536
                          tunnel: [w551 w556 w561] -> w535
                          tunnel: w537 -> [w550 w555 w560]
                          tunnel: w538 -> [w549 w554 w559]
                          frame 0 {
                            n123 = property class="Instr"(reference=w550, error in=w549) -> (reference out=w552:refnum<visa-resource-name>, error out=w553:errorcluster, "Bytes at Port"=w551:u32)
                          }
                          frame 1.. {
                            n124 = property class="Instr"(reference=w555, error in=w554) -> (reference out=w557:refnum<visa-resource-name>, error out=w558:errorcluster, "Bytes at Port"=w556:u32)
                          }
                          frame Default {
                          }
                        }
                        n125 = Wait (ms)(milliseconds to wait=w544) -> ()  [unwired: 1 out]
                        n126 = Divide(x=w539, y=w544) -> (x/y=w543:dbl)
                        n127 = To Long Integer(number=w543) -> (32bit integer=w542:i32)
                        n128 = Greater?(x=w531, y=w542) -> (0:w541:bool)
                        n129 = VISA Read(VISA resource name=w536, byte count=w535, error in (no error)=w534) -> (VISA resource name out=w546:refnum<visa-resource-name>, read buffer=w527:string, return count=w526:u32, error out=w545:errorcluster)
                        n130 = Match Pattern(string=w527, regular expression=w529) -> (match substring=w528:string)  [unwired: 1 in, 3 out]
                        n131 = Empty String/Path?(string/path=w528) -> (empty?=w530:bool)
                        n132 = Not Equal?(x=w529, y="null") -> (x != y?=w547:bool)
                        n133 = case shown="True" w547 {
                          tunnel: [TRUE w563] -> w540
                          tunnel: w530 -> [_ w564]
                          frame False {
                          }
                          frame True {
                            n134 = case shown="False" w564 {
                              tunnel: [FALSE TRUE] -> w563
                              frame True {
                              }
                              frame False {
                              }
                            }
                          }
                        }
                        n135 = local write "Dreply"(w527) -> ()
                        n136 = local write "Dbytes out"(w526) -> ()
                        n137 = Or(x=w540, y=w541) -> (x .or. y?=w532:bool)
                      }
                    }
                  }
                }
              }
            }
            frame "Ludl_Kinetec" {
              n138 = case shown="Default" w571 {
                tunnel: [w579 w675 w863] -> w577
                tunnel: w576 -> [w580 w676 w864]
                tunnel: w575 -> [w583 w679 w867]
                tunnel: w574 -> [w581 w677 w865]
                tunnel: [w578 w674 w862] -> w573
                tunnel: w572 -> [w582 w678 w866]
                tunnel: w570 -> [_ w671 _]
                tunnel: w569 -> [w584 w680 w868]
                tunnel: w568 -> [_ w673 _]
                tunnel: w567 -> [_ w672 _]
                frame Default {
                  n139 = disable-structure shown="Enabled" {
                    disable-tunnel: w584 -> [w591 _]
                    disable-tunnel: w583 -> [w590 _]
                    disable-tunnel: w582 -> [w589 _]
                    disable-tunnel: w581 -> [w588 w670]
                    disable-tunnel: w580 -> [w587 _]
                    disable-tunnel: [w586 w670] -> w579
                    disable-tunnel: [w585 "" ("read buffer")] -> w578
                    frame Enabled {
                      # "home XYZ"
                      # "target XYZ"
                      n140 = while {
                        shift-right: [w600] -> _
                        shift-left: w590 -> [w598]
                        shift-right: [w601] -> w586
                        shift-left: w588 -> [w596]
                        tunnel: w587 -> [w595]
                        tunnel: [w602] -> w585
                        tunnel: w591 -> [w599]
                        tunnel: w589 -> [w597]
                        i -> [w594]
                        stop <- w603 stop-if-true
                        n141 = flat-sequence {
                          tunnel: w598 -> [w616]
                          tunnel: w596 -> [w617]
                          tunnel: w595 -> [w619]
                          tunnel: [w619] -> w611
                          tunnel: [w613] -> w610
                          tunnel: [w614] -> w609
                          tunnel: [w618] -> w608
                          tunnel: w599 -> [w615]
                          tunnel: w597 -> [w614]
                          tunnel: w594 -> [w612]
                          tunnel: [w612] -> w592
                          tunnel: [w625] -> w607
                          tunnel: [w624] -> w606
                          tunnel: [w623] -> w605
                          tunnel: [w622] -> w604
                          tunnel: w611 -> [w625]
                          tunnel: w610 -> [w623]
                          tunnel: w609 -> [w622]
                          tunnel: w608 -> [w624]
                          tunnel: [w620] -> w593
                          tunnel: w592 -> [w620]
                          tunnel: [w646] -> w600
                          tunnel: [w645] -> w601
                          tunnel: [w627] -> w602
                          tunnel: w607 -> [w629]
                          tunnel: w606 -> [w638]
                          tunnel: w605 -> [w637]
                          tunnel: w604 -> [w633]
                          tunnel: [w632] -> w603
                          tunnel: w593 -> [w631]
                          frame #0 {
                            # "target XYZ"
                            n142 = VISA Write(VISA resource name=w616, write buffer=w615, error in (no error)=w617) -> (VISA resource name out=w613:refnum<visa-resource-name>, error out=w618:errorcluster)  [unwired: 1 out]
                          }
                          frame #1 {
                            n143 = local read "delay"() -> (w621:u32)
                            n144 = Wait (ms)(milliseconds to wait=w621) -> ()  [unwired: 1 out]
                          }
                          frame #2 {
                            w644 = u32 10 ("milliseconds to wait")
                            n145 = local read "timeout"() -> (w639:i32)
                            n146 = case shown="Default" w633 {
                              selector: w633 -> [_ _ w661]
                              tunnel: [w653 w658 w659] -> w634
                              tunnel: [w652 w657 w660] -> w636
                              tunnel: [w651 w656 w661] -> w635
                              tunnel: w637 -> [w650 w655 w660]
                              tunnel: w638 -> [w649 w654 w659]
                              frame 0 {
                                n147 = property class="Instr"(reference=w650, error in=w649) -> (reference out=w652:refnum<visa-resource-name>, error out=w653:errorcluster, "Bytes at Port"=w651:u32)
                              }
                              frame 1.. {
                                n148 = property class="Instr"(reference=w655, error in=w654) -> (reference out=w657:refnum<visa-resource-name>, error out=w658:errorcluster, "Bytes at Port"=w656:u32)
                              }
                              frame Default {
                              }
                            }
                            n149 = Wait (ms)(milliseconds to wait=w644) -> ()  [unwired: 1 out]
                            n150 = Divide(x=w639, y=w644) -> (x/y=w643:dbl)
                            n151 = To Long Integer(number=w643) -> (32bit integer=w642:i32)
                            n152 = Greater?(x=w631, y=w642) -> (0:w641:bool)
                            n153 = VISA Read(VISA resource name=w636, byte count=w635, error in (no error)=w634) -> (VISA resource name out=w646:refnum<visa-resource-name>, read buffer=w627:string, return count=w626:u32, error out=w645:errorcluster)
                            n154 = Match Pattern(string=w627, regular expression=w629) -> (match substring=w628:string)  [unwired: 1 in, 3 out]
                            n155 = Empty String/Path?(string/path=w628) -> (empty?=w630:bool)
                            n156 = Not Equal?(x=w629, y="null") -> (x != y?=w647:bool)
                            n157 = case shown="True" w647 {
                              tunnel: [TRUE w663] -> w640
                              tunnel: w630 -> [_ w664]
                              frame False {
                              }
                              frame True {
                                n158 = case shown="False" w664 {
                                tunnel: [FALSE TRUE] -> w663
                                frame True {
                                }
                                frame False {
                                }
                                }
                              }
                            }
                            n159 = local write "Dreply"(w627) -> ()
                            n160 = local write "Dbytes out"(w626) -> ()
                            n161 = Or(x=w640, y=w641) -> (x .or. y?=w632:bool)
                          }
                        }
                      }
                    }
                    frame Disabled {
                      n162 = local write "Dreply"("Default" ("Dreply")) -> ()
                      n163 = local write "Dbytes out"(u32 0 ("Dbytes out")) -> ()
                    }
                  }
                }
                frame "XY-STAGE:MOVE" {
                  n164 = stacked-sequence {
                    seq-local: [w681 _ _] -> [_ w779 _]
                    seq-local: [_ w778 _] -> [_ _ w782]
                    seq-local: [w682 _ _] -> [_ w777 _]
                    seq-local: [_ w776 _] -> [_ _ w780]
                    tunnel: w680 -> [_ _ w786]
                    tunnel: w679 -> [w692 _ _]
                    tunnel: w678 -> [w691 _ w785]
                    tunnel: w677 -> [w690 _ _]
                    tunnel: w676 -> [w689 _ w784]
                    tunnel: [_ _ w781] -> w675
                    tunnel: [_ _ w783] -> w674
                    tunnel: w673 -> [w686 _ _]
                    tunnel: w672 -> [w685 _ _]
                    tunnel: w671 -> [w683 _ _]
                    frame #0 {
                      n165 = Not Equal To 0?(x=w686) -> (x != 0?=w688:bool)
                      n166 = Not Equal To 0?(x=w685) -> (x != 0?=w687:bool)
                      n167 = Or(x=w688, y=w687) -> (x .or. y?=w684:bool)
                      n168 = case shown="True" w684 {
                        tunnel: w692 -> [w694 w701]
                        tunnel: w691 -> [_ w700]
                        tunnel: w690 -> [w693 w699]
                        tunnel: w689 -> [_ w698]
                        tunnel: [w693 w697] -> w682
                        tunnel: w683 -> [_ w696]
                        tunnel: [w694 w695] -> w681
                        frame False {
                        }
                        frame True {
                          # "home XYZ"
                          n169 = while {
                            shift-right: [w710] -> w695
                            shift-left: w701 -> [w709]
                            shift-right: [w711] -> w697
                            shift-left: w699 -> [w707]
                            tunnel: w698 -> [w706]
                            tunnel: w700 -> [w708]
                            tunnel: w696 -> [w702]
                            i -> [w705]
                            stop <- w712 stop-if-true
                            n170 = flat-sequence {
                              tunnel: w709 -> [w725]
                              tunnel: w707 -> [w726]
                              tunnel: w706 -> [w728]
                              tunnel: [w728] -> w720
                              tunnel: [w723] -> w719
                              tunnel: [w724] -> w718
                              tunnel: [w727] -> w717
                              tunnel: w708 -> [w724]
                              tunnel: w705 -> [w722]
                              tunnel: [w722] -> w703
                              tunnel: w702 -> [w721]
                              tunnel: [w734] -> w716
                              tunnel: [w733] -> w715
                              tunnel: [w732] -> w714
                              tunnel: [w731] -> w713
                              tunnel: w720 -> [w734]
                              tunnel: w719 -> [w732]
                              tunnel: w718 -> [w731]
                              tunnel: w717 -> [w733]
                              tunnel: [w729] -> w704
                              tunnel: w703 -> [w729]
                              tunnel: [w755] -> w710
                              tunnel: [w754] -> w711
                              tunnel: w716 -> [w738]
                              tunnel: w715 -> [w747]
                              tunnel: w714 -> [w746]
                              tunnel: w713 -> [w742]
                              tunnel: [w741] -> w712
                              tunnel: w704 -> [w740]
                              frame #0 {
                                # "home XYZ"
                                n171 = VISA Write(VISA resource name=w725, write buffer=w721, error in (no error)=w726) -> (VISA resource name out=w723:refnum<visa-resource-name>, error out=w727:errorcluster)  [unwired: 1 out]
                              }
                              frame #1 {
                                n172 = local read "delay"() -> (w730:u32)
                                n173 = Wait (ms)(milliseconds to wait=w730) -> ()  [unwired: 1 out]
                              }
                              frame #2 {
                                w753 = u32 10 ("milliseconds to wait")
                                n174 = local read "timeout"() -> (w748:i32)
                                n175 = case shown="Default" w742 {
                                selector: w742 -> [_ _ w770]
                                tunnel: [w762 w767 w768] -> w743
                                tunnel: [w761 w766 w769] -> w745
                                tunnel: [w760 w765 w770] -> w744
                                tunnel: w746 -> [w759 w764 w769]
                                tunnel: w747 -> [w758 w763 w768]
                                frame 0 {
                                n176 = property class="Instr"(reference=w759, error in=w758) -> (reference out=w761:refnum<visa-resource-name>, error out=w762:errorcluster, "Bytes at Port"=w760:u32)
                                }
                                frame 1.. {
                                n177 = property class="Instr"(reference=w764, error in=w763) -> (reference out=w766:refnum<visa-resource-name>, error out=w767:errorcluster, "Bytes at Port"=w765:u32)
                                }
                                frame Default {
                                }
                                }
                                n178 = Wait (ms)(milliseconds to wait=w753) -> ()  [unwired: 1 out]
                                n179 = Divide(x=w748, y=w753) -> (x/y=w752:dbl)
                                n180 = To Long Integer(number=w752) -> (32bit integer=w751:i32)
                                n181 = Greater?(x=w740, y=w751) -> (0:w750:bool)
                                n182 = VISA Read(VISA resource name=w745, byte count=w744, error in (no error)=w743) -> (VISA resource name out=w755:refnum<visa-resource-name>, read buffer=w736:string, return count=w735:u32, error out=w754:errorcluster)
                                n183 = Match Pattern(string=w736, regular expression=w738) -> (match substring=w737:string)  [unwired: 1 in, 3 out]
                                n184 = Empty String/Path?(string/path=w737) -> (empty?=w739:bool)
                                n185 = Not Equal?(x=w738, y="null") -> (x != y?=w756:bool)
                                n186 = case shown="True" w756 {
                                tunnel: [TRUE w772] -> w749
                                tunnel: w739 -> [_ w773]
                                frame False {
                                }
                                frame True {
                                n187 = case shown="False" w773 {
                                tunnel: [FALSE TRUE] -> w772
                                frame True {
                                }
                                frame False {
                                }
                                }
                                }
                                }
                                n188 = local write "Dreply"(w736) -> ()
                                n189 = local write "Dbytes out"(w735) -> ()
                                n190 = Or(x=w749, y=w750) -> (x .or. y?=w741:bool)
                              }
                            }
                          }
                        }
                      }
                    }
                    frame #1 {
                      n191 = call "XYZ_XYStage_Status.vi"("error in (no error)"=w777, "VISA resource name"=w779) -> ("error out"=w776:errorcluster, "VISA resource name out"=w778:refnum<visa-resource-name>)  [unwired: 4 in, 1 out]
                    }
                    frame #2 {
                      # "target XYZ"
                      n192 = while {
                        shift-right: [w795] -> _
                        shift-left: w782 -> [w793]
                        shift-right: [w796] -> w781
                        shift-left: w780 -> [w791]
                        tunnel: w784 -> [w790]
                        tunnel: [w797] -> w783
                        tunnel: w786 -> [w794]
                        tunnel: w785 -> [w792]
                        i -> [w789]
                        stop <- w798 stop-if-true
                        n193 = flat-sequence {
                          tunnel: w793 -> [w811]
                          tunnel: w791 -> [w812]
                          tunnel: w790 -> [w814]
                          tunnel: [w814] -> w806
                          tunnel: [w809] -> w805
                          tunnel: [w810] -> w804
                          tunnel: [w813] -> w803
                          tunnel: w794 -> [w807]
                          tunnel: w792 -> [w810]
                          tunnel: w789 -> [w808]
                          tunnel: [w808] -> w787
                          tunnel: [w820] -> w802
                          tunnel: [w819] -> w801
                          tunnel: [w818] -> w800
                          tunnel: [w817] -> w799
                          tunnel: w806 -> [w820]
                          tunnel: w805 -> [w818]
                          tunnel: w804 -> [w817]
                          tunnel: w803 -> [w819]
                          tunnel: [w815] -> w788
                          tunnel: w787 -> [w815]
                          tunnel: [w841] -> w795
                          tunnel: [w840] -> w796
                          tunnel: [w822] -> w797
                          tunnel: w802 -> [w824]
                          tunnel: w801 -> [w833]
                          tunnel: w800 -> [w832]
                          tunnel: w799 -> [w828]
                          tunnel: [w827] -> w798
                          tunnel: w788 -> [w826]
                          frame #0 {
                            # "target XYZ"
                            n194 = VISA Write(VISA resource name=w811, write buffer=w807, error in (no error)=w812) -> (VISA resource name out=w809:refnum<visa-resource-name>, error out=w813:errorcluster)  [unwired: 1 out]
                          }
                          frame #1 {
                            n195 = local read "delay"() -> (w816:u32)
                            n196 = Wait (ms)(milliseconds to wait=w816) -> ()  [unwired: 1 out]
                          }
                          frame #2 {
                            w839 = u32 10 ("milliseconds to wait")
                            n197 = local read "timeout"() -> (w834:i32)
                            n198 = case shown="Default" w828 {
                              selector: w828 -> [_ _ w856]
                              tunnel: [w848 w853 w854] -> w829
                              tunnel: [w847 w852 w855] -> w831
                              tunnel: [w846 w851 w856] -> w830
                              tunnel: w832 -> [w845 w850 w855]
                              tunnel: w833 -> [w844 w849 w854]
                              frame 0 {
                                n199 = property class="Instr"(reference=w845, error in=w844) -> (reference out=w847:refnum<visa-resource-name>, error out=w848:errorcluster, "Bytes at Port"=w846:u32)
                              }
                              frame 1.. {
                                n200 = property class="Instr"(reference=w850, error in=w849) -> (reference out=w852:refnum<visa-resource-name>, error out=w853:errorcluster, "Bytes at Port"=w851:u32)
                              }
                              frame Default {
                              }
                            }
                            n201 = Wait (ms)(milliseconds to wait=w839) -> ()  [unwired: 1 out]
                            n202 = Divide(x=w834, y=w839) -> (x/y=w838:dbl)
                            n203 = To Long Integer(number=w838) -> (32bit integer=w837:i32)
                            n204 = Greater?(x=w826, y=w837) -> (0:w836:bool)
                            n205 = VISA Read(VISA resource name=w831, byte count=w830, error in (no error)=w829) -> (VISA resource name out=w841:refnum<visa-resource-name>, read buffer=w822:string, return count=w821:u32, error out=w840:errorcluster)
                            n206 = Match Pattern(string=w822, regular expression=w824) -> (match substring=w823:string)  [unwired: 1 in, 3 out]
                            n207 = Empty String/Path?(string/path=w823) -> (empty?=w825:bool)
                            n208 = Not Equal?(x=w824, y="null") -> (x != y?=w842:bool)
                            n209 = case shown="True" w842 {
                              tunnel: [TRUE w858] -> w835
                              tunnel: w825 -> [_ w859]
                              frame False {
                              }
                              frame True {
                                n210 = case shown="False" w859 {
                                tunnel: [FALSE TRUE] -> w858
                                frame True {
                                }
                                frame False {
                                }
                                }
                              }
                            }
                            n211 = local write "Dreply"(w822) -> ()
                            n212 = local write "Dbytes out"(w821) -> ()
                            n213 = Or(x=w835, y=w836) -> (x .or. y?=w827:bool)
                          }
                        }
                      }
                    }
                  }
                }
                frame "XY-STAGE:STATUS" {
                  # "home XYZ"
                  # "target XYZ"
                  n214 = while {
                    shift-right: [w877] -> _
                    shift-left: w867 -> [w875]
                    shift-right: [w878] -> w863
                    shift-left: w865 -> [w873]
                    tunnel: w864 -> [w872]
                    tunnel: [w879] -> w862
                    tunnel: w868 -> [w876]
                    tunnel: w866 -> [w874]
                    i -> [w871]
                    stop <- w880 stop-if-true
                    n215 = flat-sequence {
                      tunnel: w875 -> [w893]
                      tunnel: w873 -> [w894]
                      tunnel: w872 -> [w896]
                      tunnel: [w896] -> w888
                      tunnel: [w890] -> w887
                      tunnel: [w891] -> w886
                      tunnel: [w895] -> w885
                      tunnel: w876 -> [w892]
                      tunnel: w874 -> [w891]
                      tunnel: w871 -> [w889]
                      tunnel: [w889] -> w869
                      tunnel: [w902] -> w884
                      tunnel: [w901] -> w883
                      tunnel: [w900] -> w882
                      tunnel: [w899] -> w881
                      tunnel: w888 -> [w902]
                      tunnel: w887 -> [w900]
                      tunnel: w886 -> [w899]
                      tunnel: w885 -> [w901]
                      tunnel: [w897] -> w870
                      tunnel: w869 -> [w897]
                      tunnel: [w923] -> w877
                      tunnel: [w922] -> w878
                      tunnel: [w904] -> w879
                      tunnel: w884 -> [w906]
                      tunnel: w883 -> [w915]
                      tunnel: w882 -> [w914]
                      tunnel: w881 -> [w910]
                      tunnel: [w909] -> w880
                      tunnel: w870 -> [w908]
                      frame #0 {
                        # "target XYZ"
                        n216 = VISA Write(VISA resource name=w893, write buffer=w892, error in (no error)=w894) -> (VISA resource name out=w890:refnum<visa-resource-name>, error out=w895:errorcluster)  [unwired: 1 out]
                      }
                      frame #1 {
                        n217 = local read "delay"() -> (w898:u32)
                        n218 = Wait (ms)(milliseconds to wait=w898) -> ()  [unwired: 1 out]
                      }
                      frame #2 {
                        w921 = u32 10 ("milliseconds to wait")
                        n219 = local read "timeout"() -> (w916:i32)
                        n220 = case shown="Default" w910 {
                          selector: w910 -> [_ _ w938]
                          tunnel: [w930 w935 w936] -> w911
                          tunnel: [w929 w934 w937] -> w913
                          tunnel: [w928 w933 w938] -> w912
                          tunnel: w914 -> [w927 w932 w937]
                          tunnel: w915 -> [w926 w931 w936]
                          frame 0 {
                            n221 = property class="Instr"(reference=w927, error in=w926) -> (reference out=w929:refnum<visa-resource-name>, error out=w930:errorcluster, "Bytes at Port"=w928:u32)
                          }
                          frame 1.. {
                            n222 = property class="Instr"(reference=w932, error in=w931) -> (reference out=w934:refnum<visa-resource-name>, error out=w935:errorcluster, "Bytes at Port"=w933:u32)
                          }
                          frame Default {
                          }
                        }
                        n223 = Wait (ms)(milliseconds to wait=w921) -> ()  [unwired: 1 out]
                        n224 = Divide(x=w916, y=w921) -> (x/y=w920:dbl)
                        n225 = To Long Integer(number=w920) -> (32bit integer=w919:i32)
                        n226 = Greater?(x=w908, y=w919) -> (0:w918:bool)
                        n227 = VISA Read(VISA resource name=w913, byte count=w912, error in (no error)=w911) -> (VISA resource name out=w923:refnum<visa-resource-name>, read buffer=w904:string, return count=w903:u32, error out=w922:errorcluster)
                        n228 = Match Pattern(string=w904, regular expression=w906) -> (match substring=w905:string)  [unwired: 1 in, 3 out]
                        n229 = Empty String/Path?(string/path=w905) -> (empty?=w907:bool)
                        n230 = Not Equal?(x=w906, y="null") -> (x != y?=w924:bool)
                        n231 = case shown="True" w924 {
                          tunnel: [TRUE w940] -> w917
                          tunnel: w907 -> [_ w941]
                          frame False {
                          }
                          frame True {
                            n232 = case shown="False" w941 {
                              tunnel: [FALSE TRUE] -> w940
                              frame True {
                              }
                              frame False {
                              }
                            }
                          }
                        }
                        n233 = local write "Dreply"(w904) -> ()
                        n234 = local write "Dbytes out"(w903) -> ()
                        n235 = Or(x=w917, y=w918) -> (x .or. y?=w909:bool)
                      }
                    }
                  }
                }
              }
            }
          }
        }
        frame #4 {
          n236 = case shown="\"XY-STAGE:WHERE\"" w948 {
            tunnel: w949 -> [_ w956]
            tunnel: w947 -> [_ w953]
            tunnel: [0.0 w952] -> w946
            frame Default {
            }
            frame "XY-STAGE:WHERE" {
              n237 = call <vilib>:"Space Constant.vi"() -> ("String"=w964:string)
              n238 = Search/Split String(string=w953, search string/char (-)=w964, offset (0)=0) -> (substring before match=w957:string, match + rest of string=w961:string)  [unwired: 1 out]
              n239 = local write "Dreply"(w957) -> ()
              n240 = call <vilib>:"Space Constant.vi"() -> ("String"=w960:string)
              n241 = Search/Split String(string=w961, search string/char (-)=w960, offset (0)=1) -> (substring before match=w954:string, match + rest of string=w955:string)  [unwired: 1 out]
              n242 = case shown="\"Ludl_Kinetec\"" w956 {
                tunnel: w955 -> [w967 w973]
                tunnel: [0.0 w969] -> w952
                frame "ASI_MS2000", Default {
                  n243 = Fract/Exp String To Number(string=w967, default (0 dbl)=0.0 ("default (0 I32)")) -> (number=w966:dbl)  [unwired: 2 in, 1 out]
                  n244 = local write "y"(w966) -> ()
                }
                frame "Ludl_Kinetec" {
                  n245 = call <vilib>:"Space Constant.vi"() -> ("String"=w972:string)
                  n246 = Search/Split String(string=w973, search string/char (-)=w972, offset (0)=1) -> (substring before match=w971:string)  [unwired: 2 out]
                  n247 = Fract/Exp String To Number(string=w971, default (0 dbl)=0.0 ("default (0 I32)")) -> (number=w969:dbl)  [unwired: 2 in, 1 out]
                  n248 = local write "y"(w969) -> ()
                }
              }
              n249 = Fract/Exp String To Number(string=w954, default (0 dbl)=0.0 ("default (0 I32)")) -> (number=w959:dbl)  [unwired: 2 in, 1 out]
              n250 = local write "x"(w959) -> ()
            }
          }
          n251 = Equal?(x=w946, y=2.0) -> (x = y?=w944:bool)
        }
        frame #5 {
          n252 = case shown="True" w975 {
            frame False {
            }
            frame True {
              n253 = Wait (ms)(milliseconds to wait=u32 0) -> ()  [unwired: 1 out]
            }
          }
        }
        frame #6 {
          n254 = local write "Success"(TRUE ("Success")) -> ()
        }
      }
    }
    frame "XY-STAGE:CLOSE" {
      n255 = flat-sequence {
        tunnel: w983 -> [w987]
        tunnel: w985 -> [w988]
        tunnel: [w988] -> w982
        tunnel: [w987] -> w981
        tunnel: w982 -> [w991]
        tunnel: w981 -> [w989]
        tunnel: [w990] -> w980
        tunnel: [w1002] -> w984
        tunnel: w980 -> [w1002]
        frame #0 {
          n256 = local write "Success"(FALSE ("Success")) -> ()
        }
        frame #1 {
          n257 = case shown="Default" w989 {
            tunnel: w991 -> [w993 w996 w999]
            tunnel: [w992 w995 w998] -> w990
            frame Default {
              n258 = global read "Global.vi" "XY-STAGE VISA resource name"() -> (w994:refnum<visa-resource-name>)
              n259 = VISA Close(VISA resource name=w994, error in (no error)=w993) -> (error out=w992:errorcluster)
            }
            frame "ASI_MS2000" {
              n260 = global read "Global.vi" "XY-STAGE VISA resource name"() -> (w997:refnum<visa-resource-name>)
              n261 = VISA Close(VISA resource name=w997, error in (no error)=w996) -> (error out=w995:errorcluster)
            }
            frame "Ludl_Kinetec" {
              n262 = global read "Global.vi" "XY-STAGE VISA resource name"() -> (w1000:refnum<visa-resource-name>)
              n263 = VISA Close(VISA resource name=w1000, error in (no error)=w999) -> (error out=w998:errorcluster)
            }
          }
        }
        frame #2 {
          n264 = local write "Success"(TRUE ("Success")) -> ()
        }
      }
    }
    frame "XY-STAGE:OPEN" {
      n265 = flat-sequence {
        tunnel: w1026 -> [w1040]
        tunnel: w1028 -> [w1041]
        tunnel: [w1041] -> w1025
        tunnel: [w1040] -> w1024
        tunnel: [w1038] -> w1022
        tunnel: w1021 -> [w1038]
        tunnel: [w1037] -> w1020
        tunnel: w1019 -> [w1037]
        tunnel: [w1036] -> w1018
        tunnel: w1017 -> [w1036]
        tunnel: [w1035] -> w1016
        tunnel: w1015 -> [w1035]
        tunnel: [w1034] -> w1014
        tunnel: w1013 -> [w1034]
        tunnel: [w1033] -> w1012
        tunnel: w1011 -> [w1033]
        tunnel: [w1032] -> w1010
        tunnel: w1009 -> [w1032]
        tunnel: [w1031] -> w1008
        tunnel: w1007 -> [w1031]
        tunnel: [w1030] -> w1006
        tunnel: w1005 -> [w1030]
        tunnel: [w1029] -> w1004
        tunnel: w1003 -> [w1029]
        tunnel: [w1052] -> w1023
        tunnel: w1024 -> [w1054]
        tunnel: w1025 -> [w1053]
        tunnel: w1022 -> [w1051]
        tunnel: w1020 -> [w1050]
        tunnel: w1018 -> [w1049]
        tunnel: w1016 -> [w1048]
        tunnel: w1014 -> [w1047]
        tunnel: w1012 -> [w1046]
        tunnel: w1010 -> [w1045]
        tunnel: w1008 -> [w1044]
        tunnel: w1006 -> [w1043]
        tunnel: w1004 -> [w1042]
        tunnel: [w1200] -> w1027
        tunnel: w1023 -> [w1200]
        frame #0 {
          n266 = local write "Success"(FALSE ("Success")) -> ()
        }
        frame #1 {
          n267 = case shown="\"ASI_MS2000\"" w1054 {
            tunnel: [w1058 w1081 w1169] -> w1052
            tunnel: w1053 -> [w1059 w1082 w1170]
            tunnel: w1051 -> [_ w1080 w1168]
            tunnel: w1050 -> [_ w1079 w1167]
            tunnel: w1049 -> [_ w1078 w1166]
            tunnel: w1048 -> [_ w1077 w1165]
            tunnel: w1047 -> [_ w1076 w1164]
            tunnel: w1046 -> [_ w1075 w1163]
            tunnel: w1045 -> [_ w1074 w1162]
            tunnel: w1044 -> [_ w1073 w1161]
            tunnel: w1043 -> [_ w1072 w1160]
            tunnel: w1042 -> [_ w1071 w1159]
            frame Default {
              n268 = global read "Global.vi" "XY-STAGE termination char\n(0xA = '\\n' = LF)"() -> (w1069:u8)
              n269 = global read "Global.vi" "XY-STAGE VISA resource name"() -> (w1062:refnum<visa-resource-name>)
              n270 = global read "Global.vi" "XY-STAGE flow control"() -> (w1064:u16)
              n271 = global read "Global.vi" "XY-STAGE baud rate"() -> (w1066:u32)
              n272 = global read "Global.vi" "XY-STAGE data bits"() -> (w1067:u16)
              n273 = global read "Global.vi" "XY-STAGE stop bits"() -> (w1065:u16)
              n274 = global read "Global.vi" "XY-STAGE parity"() -> (w1068:enum16{"None", "Odd", "Even", "Mark", "Space"})
              n275 = call-poly "VISA Configure Serial Port"("VISA resource name"=w1062, "termination char\n(0xA = '\\n' = LF)"=w1069, "baud rate (9600)"=w1066, "data bits (8)"=w1067, "parity (0:none)"=w1068, "error in (no error)"=w1059, "stop bits (10: 1 bit)"=w1065, "flow control (0:none)"=w1064) -> ("VISA resource name out"=w1070:refnum<visa-resource-name>, "error out"=w1055:errorcluster)  [unwired: 6 in]
              n276 = global read "Global.vi" "XY-STAGE mask"() -> (w1063:u16)
              n277 = Unbundle By Name(w1055) -> ("status"=w1056:bool)
              n278 = Stop(stop? (T)=w1056) -> ()
              n279 = VISA Flush I/O Buffer(VISA resource name=w1070, mask (16)=w1063, error in (no error)=w1055) -> (VISA resource name out=w1061:refnum<visa-resource-name>, error out=w1057:errorcluster)
              n280 = global read "Global.vi" "XY-STAGE maskT"() -> (w1060:u16)
              n281 = VISA Flush I/O Buffer(VISA resource name=w1061, mask (16)=w1060, error in (no error)=w1057) -> (error out=w1058:errorcluster)  [unwired: 1 out]
            }
            frame "ASI_MS2000" {
              n282 = flat-sequence {
                tunnel: [w1096] -> w1081
                tunnel: w1082 -> [w1095]
                tunnel: w1080 -> [w1092]
                tunnel: w1079 -> [w1091]
                tunnel: w1078 -> [w1090]
                tunnel: w1077 -> [w1089]
                tunnel: w1076 -> [w1088]
                tunnel: w1075 -> [w1087]
                tunnel: w1074 -> [w1086]
                tunnel: w1073 -> [w1085]
                tunnel: w1072 -> [w1084]
                tunnel: w1071 -> [w1083]
                frame #0 {
                  n283 = call-poly "VISA Configure Serial Port"("VISA resource name"=w1089, "timeout (10sec)"=w1090, "termination char\n(0xA = '\\n' = LF)"=w1091, "Enable Termination\nChar (T)"=w1092, "baud rate (9600)"=w1088, "data bits (8)"=w1087, "parity (0:none)"=w1086, "error in (no error)"=w1095, "stop bits (10: 1 bit)"=w1085, "flow control (0:none)"=w1084) -> ("VISA resource name out"=w1099:refnum<visa-resource-name>, "error out"=w1097:errorcluster)  [unwired: 4 in]
                  n284 = Unbundle By Name(w1097) -> ("status"=w1098:bool)
                  n285 = Stop(stop? (T)=w1098) -> ()
                  n286 = for {
                    shift-right: [w1101] -> w1093
                    shift-left: w1099 -> [w1104]
                    shift-right: [w1102] -> w1094
                    shift-left: w1097 -> [w1103]
                    tunnel: w1083 -> [w1100] mode=indexing
                    # "Flush Buffer loop"
                    n287 = VISA Flush I/O Buffer(VISA resource name=w1104, mask (16)=w1100, error in (no error)=w1103) -> (VISA resource name out=w1101:refnum<visa-resource-name>, error out=w1102:errorcluster)
                  }
                  n288 = disable-structure shown="Enabled" {
                    disable-tunnel: w1094 -> [w1107 w1158]
                    disable-tunnel: w1093 -> [w1106 _]
                    disable-tunnel: [w1105 w1158] -> w1096
                    frame Enabled {
                      n289 = flat-sequence {
                        tunnel: w1106 -> [w1115]
                        tunnel: w1107 -> [w1116]
                        tunnel: [w1116] -> w1113
                        tunnel: [w1115] -> w1112
                        tunnel: w1113 -> [w1121]
                        tunnel: w1112 -> [w1120]
                        tunnel: [w1118] -> w1111
                        tunnel: [w1117] -> w1110
                        tunnel: w1111 -> [w1129]
                        tunnel: w1110 -> [w1131]
                        tunnel: [w1128] -> w1109
                        tunnel: [w1130] -> w1108
                        tunnel: [w1142] -> w1105
                        tunnel: w1109 -> [w1143]
                        tunnel: w1108 -> [w1141]
                        frame #0 {
                          n290 = Wait (ms)(milliseconds to wait=u32 100) -> ()  [unwired: 1 out]
                        }
                        frame #1 {
                          # "initialize as needed"
                          # "PCROS X? Y? Z? (firmware settings)\nX=0.000024 Y=0.000024 Z=0.000055"
                          n291 = disable-structure shown="Enabled" {
                            disable-tunnel: [w1122 w1125] -> w1119
                            frame Disabled {
                              n292 = global read "Global.vi" "XY-STAGE command terminator"() -> (w1124:string)
                              n293 = Concatenate Strings("PCROS Z=0.000075" ("string"), w1124) -> (w1122:string)
                            }
                            frame Enabled {
                              n294 = global read "Global.vi" "XY-STAGE command terminator"() -> (w1127:string)
                              n295 = Concatenate Strings("I Z" ("string"), w1127) -> (w1125:string)
                            }
                          }
                          n296 = VISA Write(VISA resource name=w1120, write buffer=w1119, error in (no error)=w1121) -> (VISA resource name out=w1117:refnum<visa-resource-name>, error out=w1118:errorcluster)  [unwired: 1 out]
                        }
                        frame #2 {
                          n297 = disable-structure shown="Enabled" {
                            disable-tunnel: w1131 -> [w1133 w1136]
                            disable-tunnel: [w1133 w1136] -> w1130
                            disable-tunnel: [w1132 w1135] -> w1128
                            disable-tunnel: w1129 -> [w1132 w1135]
                            frame Enabled {
                              n298 = Wait (ms)(milliseconds to wait=u32 1000) -> ()  [unwired: 1 out]
                            }
                            frame Disabled {
                            }
                          }
                        }
                        frame #3 {
                          w1140 = ""
                          w1139 = 0
                          n299 = local write "Dreply"(w1140) -> ()
                          n300 = local write "Dbytes out"(w1139) -> ()
                          n301 = while {
                            tunnel: w1143 -> [w1157]
                            tunnel: [w1156] -> w1142
                            tunnel: w1141 -> [w1155]
                            shift-right: [w1148] -> w1138
                            shift-left: w1140 -> [w1149]
                            shift-right: [w1147] -> w1137
                            shift-left: w1139 -> [w1146]
                            stop <- w1150 stop-if-true
                            n302 = property class="Instr"(reference=w1155, error in=w1157) -> (reference out=w1153:refnum<visa-resource-name>, error out=w1154:errorcluster, "Bytes at Port"=w1151:u32)
                            n303 = Wait (ms)(milliseconds to wait=u32 50) -> ()  [unwired: 1 out]
                            n304 = VISA Read(VISA resource name=w1153, byte count=w1151, error in (no error)=w1154) -> (read buffer=w1145:string, return count=w1144:u32, error out=w1156:errorcluster)  [unwired: 1 out]
                            n305 = Add(x=w1146, y=w1144) -> (x+y=w1147:u32)
                            n306 = Concatenate Strings(w1149, w1145) -> (w1148:string)
                            n307 = Equal To 0?(x=w1151) -> (x = 0?=w1150:bool)
                          }
                          n308 = local write "Dreply"(w1138) -> ()
                          n309 = local write "Dbytes out"(w1137) -> ()
                        }
                      }
                    }
                    frame Disabled {
                    }
                  }
                }
              }
            }
            frame "Ludl_Kinetec" {
              n310 = flat-sequence {
                tunnel: [w1173] -> w1169
                tunnel: w1170 -> [w1190]
                tunnel: w1168 -> [w1189]
                tunnel: w1167 -> [w1188]
                tunnel: w1166 -> [w1187]
                tunnel: w1165 -> [w1186]
                tunnel: w1164 -> [w1185]
                tunnel: w1163 -> [w1184]
                tunnel: w1162 -> [w1183]
                tunnel: w1161 -> [w1182]
                tunnel: w1160 -> [w1181]
                tunnel: w1159 -> [w1180]
                frame #0 {
                  n311 = call-poly "VISA Configure Serial Port"("VISA resource name"=w1186, "timeout (10sec)"=w1187, "termination char\n(0xA = '\\n' = LF)"=w1188, "Enable Termination\nChar (T)"=w1189, "baud rate (9600)"=w1185, "data bits (8)"=w1184, "parity (0:none)"=w1183, "error in (no error)"=w1190, "stop bits (10: 1 bit)"=w1182, "flow control (0:none)"=w1181) -> ("VISA resource name out"=w1193:refnum<visa-resource-name>, "error out"=w1191:errorcluster)  [unwired: 4 in]
                  n312 = Unbundle By Name(w1191) -> ("status"=w1192:bool)
                  n313 = Stop(stop? (T)=w1192) -> ()
                  n314 = for {
                    shift-right: [w1195] -> w1172
                    shift-left: w1193 -> [w1198]
                    shift-right: [w1196] -> w1174
                    shift-left: w1191 -> [w1197]
                    tunnel: w1180 -> [w1194] mode=indexing
                    # "Flush Buffer loop"
                    n315 = VISA Flush I/O Buffer(VISA resource name=w1198, mask (16)=w1194, error in (no error)=w1197) -> (VISA resource name out=w1195:refnum<visa-resource-name>, error out=w1196:errorcluster)
                  }
                  n316 = Byte Array To String(unsigned byte array=u8[] [255]) -> (string=w1176:string)
                  n317 = Byte Array To String(unsigned byte array=u8[] [65]) -> (string=w1178:string)
                  n318 = Concatenate Strings(w1176, w1178, "\\n") -> (w1171:string)
                  n319 = VISA Write(VISA resource name=w1172, write buffer=w1171, error in (no error)=w1174) -> (error out=w1173:errorcluster)  [unwired: 2 out]
                }
              }
            }
          }
        }
        frame #2 {
          n320 = local write "Success"(TRUE ("Success")) -> ()
        }
      }
    }
  }
  n321 = call <vilib>:"Simple Error Handler.vi"("error in (no error)"=w45) -> ("error out"=→"Error out":errorcluster)  [unwired: 1 in, 7 out]
